vi "Account_Manager.vi"(11 "connection reference":T1) -> ()   [LabVIEW 2015]
uses:
  <vilib>/addons/database/Connection.llb/Conn ObjectReference.ctl
  <vilib>/addons/database/Connection.llb/Conn Execute.vi
  <vilib>/addons/database/Recordset.llb/Rec Destroy - Connection.vi
  <vilib>/addons/database/_DB Variant To Data/Database Variant To Data.xnode
  <vilib>/addons/database/NI_Database_API.lvlib
  <vilib>/addons/database/Connection.llb/DB Tools Open Connec (String).vi
panel:
  in  "Name":string
  out "Acount Access":string[][](table)
  in  "Close Button":bool
  in  "Remove Button":bool
  in  "Add Button":bool
  in  "Level":string(combo)="User"
  in  "Password":string
  in  "Ecode":string
  # "ACCOUNT MANAGEMENT"
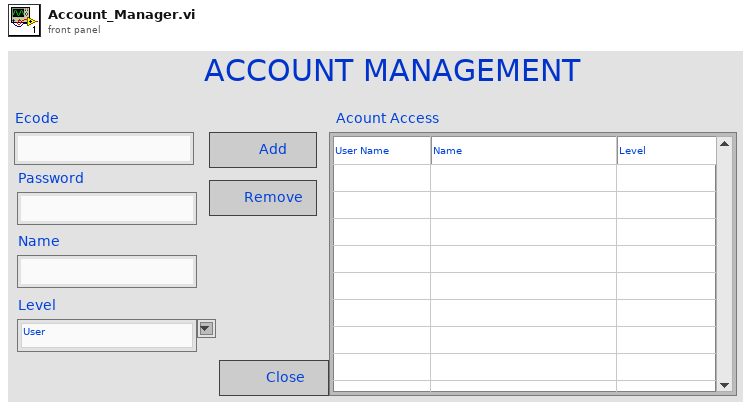
[diagram p1: front panel]
types:
  T1 = typedef "NI_Database_API.lvlib/Conn ObjectReference.ctl" = refnum<k1>
  T2 = typedef "NI_Database_API.lvlib/Rec ObjectReference.ctl" = refnum<k1>
  T3 = cluster{"Password":string, "Name":string, "Level":string}
  T4 = cluster{"Ecode":string, "Password":string, "Name":string, "Level":string}
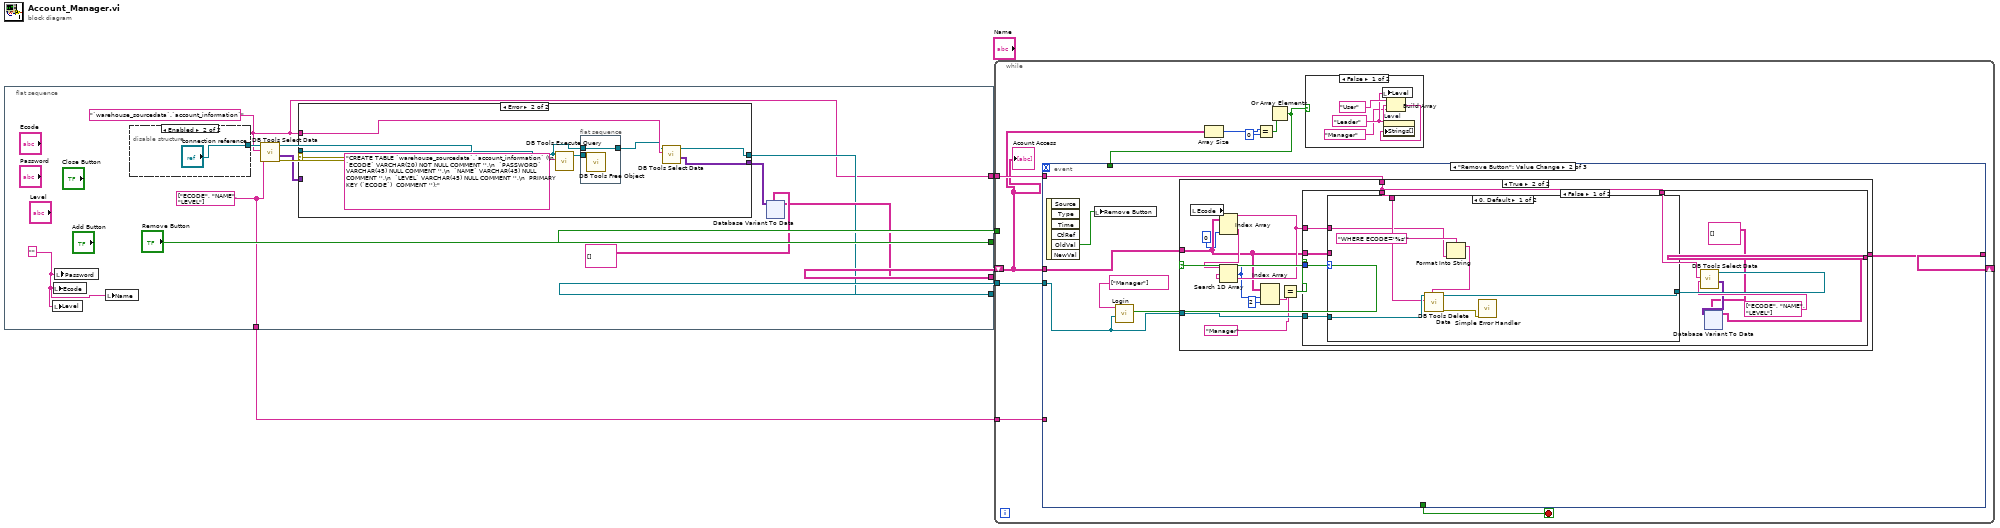
[diagram p0: block diagram]
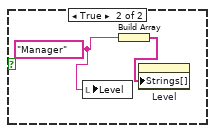
[diagram p2: hidden frame]
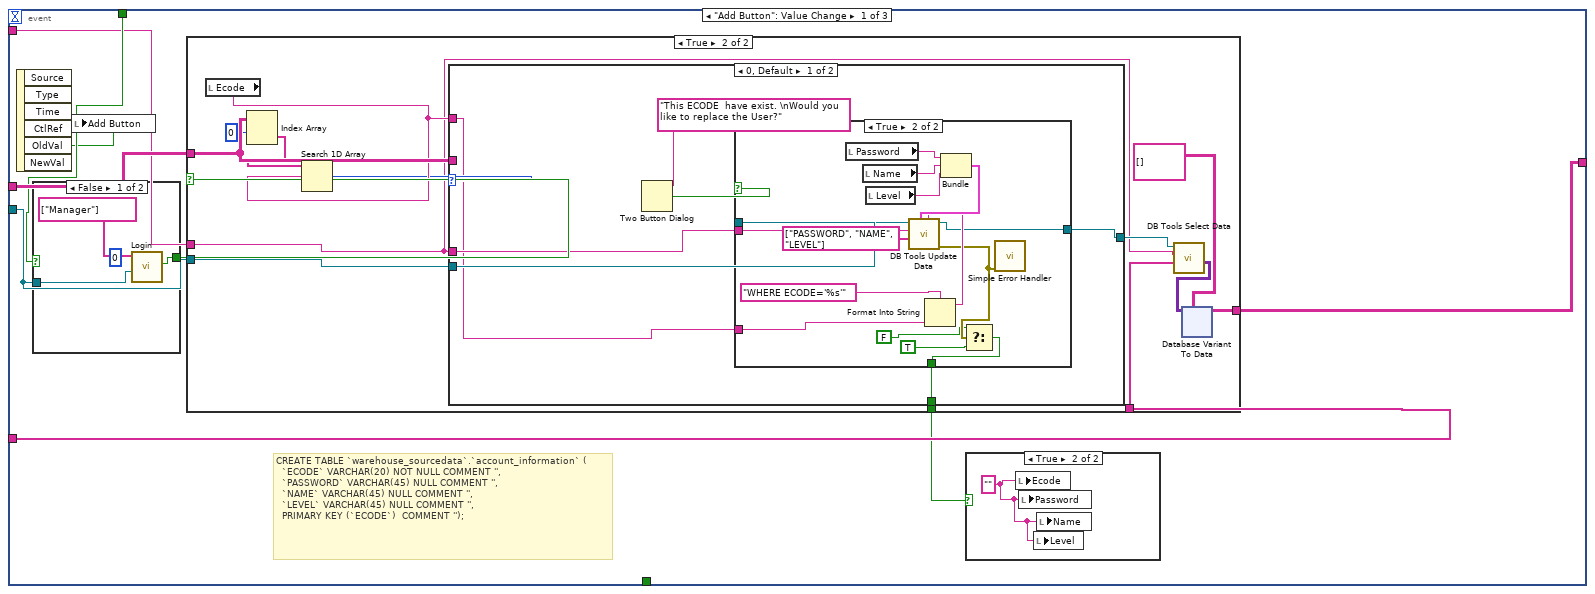
[diagram p3: hidden frame]
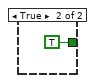
[diagram p5: hidden frame]
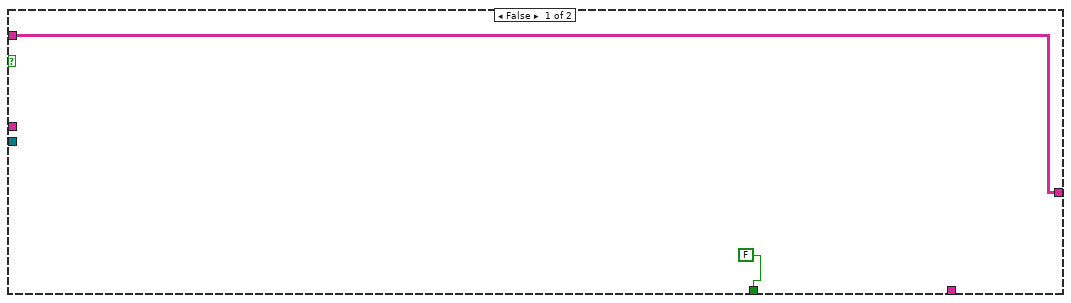
[diagram p6: hidden frame]
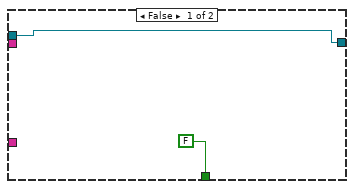
[diagram p7: hidden frame]
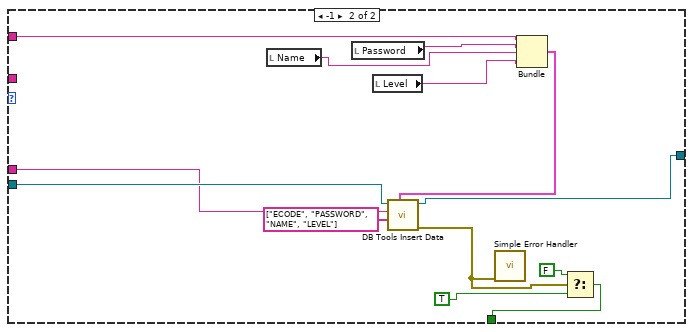
[diagram p8: hidden frame]
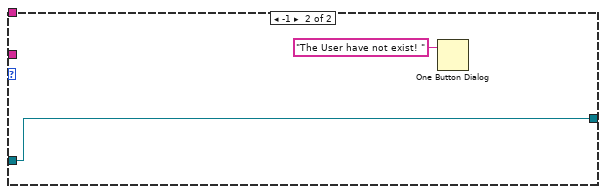
[diagram p10: hidden frame]
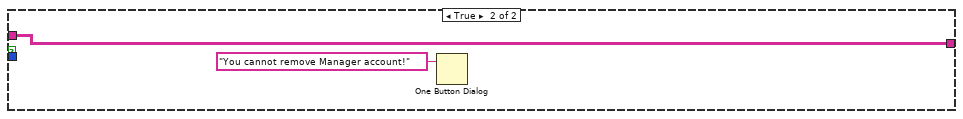
[diagram p11: hidden frame]
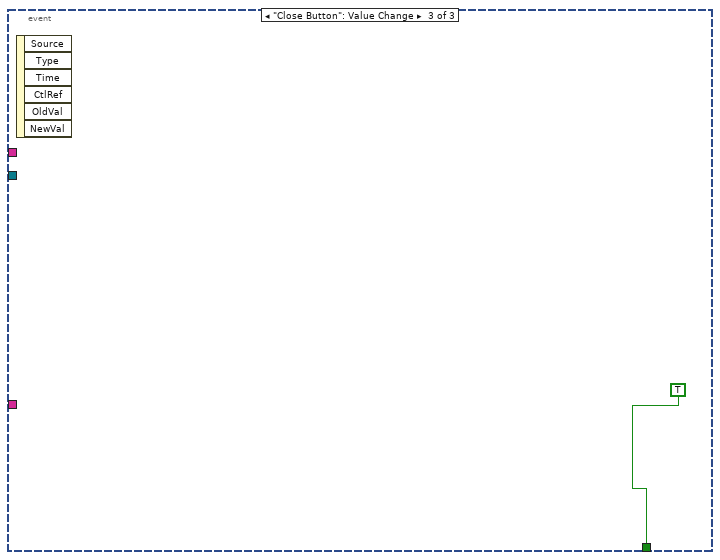
[diagram p12: hidden frame]
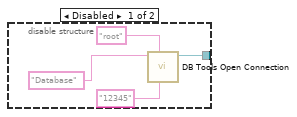
[diagram p13: hidden frame]
diagram:
  n1 = flat-sequence {
    tunnel: ["Remove Button"] -> w5
    tunnel: [w9] -> w4
    tunnel: [w10] -> w3
    tunnel: [w8] -> w2
    tunnel: [w7] -> w1
    frame #0 {
      w6 = ""
      w7 = string[] ["ECODE", "NAME", "LEVEL"] ("columns")
      w8 = "`warehouse_sourcedata`.`account_information`" ("userID")
      n2 = local write "Level"(w6) -> ()
      n3 = local write "Ecode"(w6) -> ()
      n4 = local write "Password"(w6) -> ()
      n5 = local write "Name"(w6) -> ()
      n6 = disable-structure shown="Enabled" {
        disable-tunnel: [w18 "connection reference"] -> w16
        frame Disabled {
          n7 = call-poly <vilib>:"DB Tools Open Connection.vi"("password"="12345" ("userID"), "userID"="root", "connection information"="Database" ("userID")) -> ("connection reference"=w18:T1)  [unwired: 5 in, 1 out]
        }
        frame Enabled {
        }
      }
      n8 = call <vilib>:"DB Tools Select Data.vi"("columns"=w7, "table"=w8, "connection reference"=w16) -> ("error out"=w15:errorcluster, "data"=w13:variant[][], "connection reference out"=w14:T1)  [unwired: 3 in]
      n9 = case shown="Error" w15 {
        tunnel: w14 -> [w68 w71]
        tunnel: [w68 w69] -> w9
        tunnel: w8 -> [_ w73]
        tunnel: [w67 w70] -> w12
        tunnel: w13 -> [w67 _]
        frame No Error {
        }
        frame Error {
          n10 = call-poly <vilib>:"DB Tools Execute Query.vi"("SQL query"="CREATE TABLE `warehouse_sourcedata`.`account_information` (\n  `ECODE` VARCHAR(20) NOT NULL COMMENT '',\n  `PASSWORD` VARCHAR(45) NULL COMMENT '',\n  `NAME` VARCHAR(45) NULL COMMENT '',\n  `LEVEL` VARCHAR(45) NULL COMMENT '',\n  PRIMARY KEY (`ECODE`)  COMMENT '');", "connection reference"=w71) -> ("recordset reference"=w74:T2)  [unwired: 6 in, 1 out]
          n11 = flat-sequence {
            tunnel: w74 -> [w77]
            tunnel: [w76] -> w72
            tunnel: w71 -> [w76]
            frame #0 {
              n12 = call-poly <vilib>:"DB Tools Free Object.vi"("recordset reference"=w77) -> ()  [unwired: 9 in, 2 out]
            }
          }
          n13 = call <vilib>:"DB Tools Select Data.vi"("table"=w73, "connection reference"=w72) -> ("data"=w70:variant[][], "connection reference out"=w69:T1)  [unwired: 4 in, 1 out]
        }
      }
      n14 = xnode "Database Variant To Data"("database variant"=w12, "type"=string[][] []) -> ("data"=w10:string[][])  [unwired: 1 in, 1 out]
    }
  }
  n15 = while {
    tunnel: w5 -> [_]
    shift-right: [w86] -> _
    shift-left: w3 -> [w79]
    tunnel: w4 -> [w87]
    tunnel: w2 -> [w80]
    tunnel: w1 -> [w78]
    stop <- w85 stop-if-true
    n16 = Array Size(array=w79) -> (size(s)=w83:i32[])
    n17 = Equal?(x=w83, y=0) -> (x = y?=w82:bool[])
    n18 = Or Array Elements(Boolean array=w82) -> (logical OR=w81:bool)
    n19 = event shown="[1] \"Remove Button\": Value Change" {
      selector: _ -> [_ _ _]
      dyn-events: _ -> [_ _ _]
      timeout: _ -> [_ _ _]
      tunnel: w79 -> [w101 w208 _]
      tunnel: w87 -> [w94 w204 _]
      tunnel: [w97 w207 _] -> w86
      tunnel: [_ _ TRUE] -> w85
      tunnel: w81 -> [w100 _ _]
      tunnel: w80 -> [w99 w206 _]
      tunnel: w78 -> [w98 _ _]
      event "Add Button": Value Change {
        # "CREATE TABLE `warehouse_sourcedata`.`account_information` (\n  `ECODE` VARCHAR(20) NOT NULL COMMENT '',\n  `PASSWORD` VARCHAR(45) NULL COMMENT '',\n  `NAME` VARCHAR(45) NULL COMMENT '',\n  `LEVEL` VARCHAR(45) NULL COMMENT '',\n  PRIMARY KEY (`ECODE`)  COMMENT '');"
        n20 = event-data() -> ("OldVal"=w95:bool)  [unwired: 1 in, 5 out]
        n21 = case shown="False" w100 {
          tunnel: [w105 TRUE ("OK")] -> w102
          tunnel: w94 -> [w104 _]
          frame False {
            (unwired) 0 ("Line")
            n22 = call "Login.vi"("connection reference"=w104, "Permission"=string[] ["Manager"]) -> ("OK"=w105:bool)  [unwired: 8 in, 1 out]
          }
          frame True {
          }
        }
        n23 = local write "Add Button"(w95) -> ()
        n24 = case shown="True" w102 {
          tunnel: w101 -> [w109 w121]
          tunnel: w94 -> [_ w122]
          tunnel: w99 -> [_ w115]
          tunnel: w98 -> [_ w114]
          tunnel: [w109 w111] -> w97
          tunnel: [FALSE w110] -> w96
          frame False {
          }
          frame True {
            n25 = local read "Ecode"() -> (w118:string)
            n26 = Index Array(array=w121, index (row)=0) -> (element=w119:string[])  [unwired: 1 in]
            n27 = Search 1D Array(1D array=w119, element=w118) -> (index of element=w117:i32)  [unwired: 1 in]
            n28 = case shown="0, Default" w117 {
              tunnel: w118 -> [w170 w199]
              tunnel: w122 -> [w172 w203]
              tunnel: w121 -> [_ _]
              tunnel: w115 -> [w171 w202]
              tunnel: [w169 w200] -> w116
              tunnel: [w167 w191] -> w110
              frame 0, Default {
                n29 = Two Button Dialog(message="This ECODE  have exist. \nWould you like to replace the User?") -> (T button?=w168:bool)  [unwired: 2 in]
                n30 = case shown="True" w168 {
                  tunnel: w172 -> [w175 w190]
                  tunnel: w171 -> [_ w189]
                  tunnel: w170 -> [_ w183]
                  tunnel: [w175 w180] -> w169
                  tunnel: [FALSE w176] -> w167
                  frame False {
                  }
                  frame True {
                    n31 = local read "Password"() -> (w188:string)
                    n32 = local read "Name"() -> (w187:string)
                    n33 = local read "Level"() -> (w186:string)
                    n34 = Format Into String(format string="WHERE ECODE='%s'" ("condition"), w183) -> (resulting string=w182:string)  [unwired: 2 in, 1 out]
                    n35 = Bundle("Password"=w188, "Name"=w187, "Level"=w186) -> (w185:T3)  [unwired: 1 in]
                    n36 = call <vilib>:"DB Tools Update Data.vi"("condition"=w182, "data"=w185, "columns"=string[] ["PASSWORD", "NAME", "LEVEL"], "table"=w189, "connection reference"=w190) -> ("error out"=w179:errorcluster, "connection reference out"=w180:T1)  [unwired: 5 in]
                    n37 = Select(t=FALSE, s=w179, f=TRUE) -> (s? t:f=w176:bool)
                    n38 = call <vilib>:"Simple Error Handler.vi"("error in (no error)"=w179) -> ()  [unwired: 4 in, 5 out]
                  }
                }
              }
              frame -1 {
                n39 = local read "Name"() -> (w197:string)
                n40 = local read "Password"() -> (w198:string)
                n41 = local read "Level"() -> (w196:string)
                n42 = Bundle("Ecode"=w199, "Password"=w198, "Name"=w197, "Level"=w196) -> (w195:T4)  [unwired: 1 in]
                n43 = call <vilib>:"DB Tools Insert Data.vi"("data"=w195, "columns"=string[] ["ECODE", "PASSWORD", "NAME", "LEVEL"], "table"=w202, "connection reference"=w203) -> ("error out"=w194:errorcluster, "connection reference out"=w200:T1)  [unwired: 6 in]
                n44 = call <vilib>:"Simple Error Handler.vi"("error in (no error)"=w194) -> ()  [unwired: 4 in, 5 out]
                n45 = Select(t=FALSE, s=w194, f=TRUE) -> (s? t:f=w191:bool)
              }
            }
            n46 = call <vilib>:"DB Tools Select Data.vi"("columns"=w114, "table"=w115, "connection reference"=w116) -> ("data"=w113:variant[][])  [unwired: 3 in, 2 out]
            n47 = xnode "Database Variant To Data"("database variant"=w113, "type"=string[][] []) -> ("data"=w111:string[][])  [unwired: 1 in, 1 out]
          }
        }
        n48 = case shown="True" w96 {
          frame False {
          }
          frame True {
            w103 = ""
            n49 = local write "Ecode"(w103) -> ()
            n50 = local write "Password"(w103) -> ()
            n51 = local write "Level"(w103) -> ()
            n52 = local write "Name"(w103) -> ()
          }
        }
      }
      event "Remove Button": Value Change {
        n53 = event-data() -> ("OldVal"=w205:bool)  [unwired: 1 in, 5 out]
        n54 = local write "Remove Button"(w205) -> ()
        n55 = call "Login.vi"("connection reference"=w204, "Permission"=string[] ["Manager"]) -> ("OK"=w209:bool)  [unwired: 8 in, 1 out]
        n56 = case shown="True" w209 {
          tunnel: w208 -> [w211 w219]
          tunnel: w204 -> [_ w223]
          tunnel: [w211 w220] -> w207
          tunnel: w206 -> [_ w213]
          frame False {
          }
          frame True {
            n57 = local read "Ecode"() -> (w221:string)
            n58 = Index Array(array=w219, index (col)=0 ("index (row)")) -> (element=w222:string[])  [unwired: 1 in]
            n59 = Search 1D Array(1D array=w222, element=w221) -> (index of element=w218:i32)  [unwired: 1 in]
            n60 = Index Array(array=w219, index (row)=w218, index (col)=2 ("disabled index (col)")) -> (element=w216:string)
            n61 = Equal?(x=w216, y="Manager") -> (x = y?=w214:bool)
            n62 = case shown="False" w214 {
              tunnel: w223 -> [w234 _]
              tunnel: w221 -> [w233 _]
              tunnel: [w224 w288] -> w220
              tunnel: w219 -> [w232 w288]
              tunnel: w218 -> [w231 _]
              tunnel: w213 -> [w230 _]
              tunnel: w213 -> [w228 _]
              frame False {
                n63 = case shown="0, Default" w231 {
                  tunnel: w233 -> [w282 _]
                  tunnel: w234 -> [w285 w286]
                  tunnel: w232 -> [_ _]
                  tunnel: w230 -> [w284 _]
                  tunnel: [w279 w286] -> w229
                  frame 0, Default {
                    n64 = Format Into String(format string="WHERE ECODE='%s'" ("condition"), w282) -> (resulting string=w281:string)  [unwired: 2 in, 1 out]
                    n65 = call <vilib>:"DB Tools Delete Data.vi"("condition"=w281, "table"=w284, "connection reference"=w285) -> ("error out"=w280:errorcluster, "connection reference out"=w279:T1)  [unwired: 7 in]
                    n66 = call <vilib>:"Simple Error Handler.vi"("error in (no error)"=w280) -> ()  [unwired: 4 in, 5 out]
                  }
                  frame -1 {
                    n67 = One Button Dialog(message="The User have not exist! ") -> ()  [unwired: 1 in, 1 out]
                  }
                }
                n68 = call <vilib>:"DB Tools Select Data.vi"("columns"=string[] ["ECODE", "NAME", "LEVEL"], "table"=w228, "connection reference"=w229) -> ("data"=w226:variant[][])  [unwired: 3 in, 2 out]
                n69 = xnode "Database Variant To Data"("database variant"=w226, "type"=string[][] []) -> ("data"=w224:string[][])  [unwired: 1 in, 1 out]
              }
              frame True {
                n70 = One Button Dialog(message="You cannot remove Manager account!") -> ()  [unwired: 1 in, 1 out]
              }
            }
          }
        }
      }
      event "Close Button": Value Change {
        n71 = event-data() -> ()  [unwired: 1 in, 6 out]
      }
    }
    n72 = case shown="False" w81 {
      frame False {
        w89 = "Leader" ("Level")
        n73 = local write "Level"(w89) -> ()
        n74 = Build Array("User" ("Level"), w89, "Manager" ("Level")) -> (w90:string[])
        n75 = property on="Level" class="CmbBox"("Strings[]"=w90) -> ()  [unwired: 2 in, 2 out]
      }
      frame True {
        w92 = "Manager" ("Level")
        n76 = local write "Level"(w92) -> ()
        n77 = Build Array(w92) -> (w93:string[])
        n78 = property on="Level" class="CmbBox"("Strings[]"=w93) -> ()  [unwired: 2 in, 2 out]
      }
    }
    "Acount Access" <- w79
  }
